vi "Przetwarzanie_szybkie_test.vi"() -> ()   [LabVIEW 2013]
uses:
  Kontrolki/Przetwarzanie/Kanaly.ctl
  Kontrolki/FVGs/FVG akwizycje akcje.ctl
  Kontrolki/FVGs/FVG akcje podstawowa.ctl
  <vilib>/measure/NI_MABase.lvlib
panel:
  in  "#cores (1)":i32=1
  out "szybka czasy":u32[](array[numeric])
  out "œrednia (ms)":dbl
  in  "stop":bool
  in  "L kanalow":i32=4
  out "Szybka":waveform(dbl)[](graph)
  in  "Szybka ZAKONCZ":bool
  out "Slide":dbl(slide)
  in  "Probki do usr":i32
  in  "#Cores (1)":i32=1
  out "# elements in queue":i32
  out "szybka czas":u32
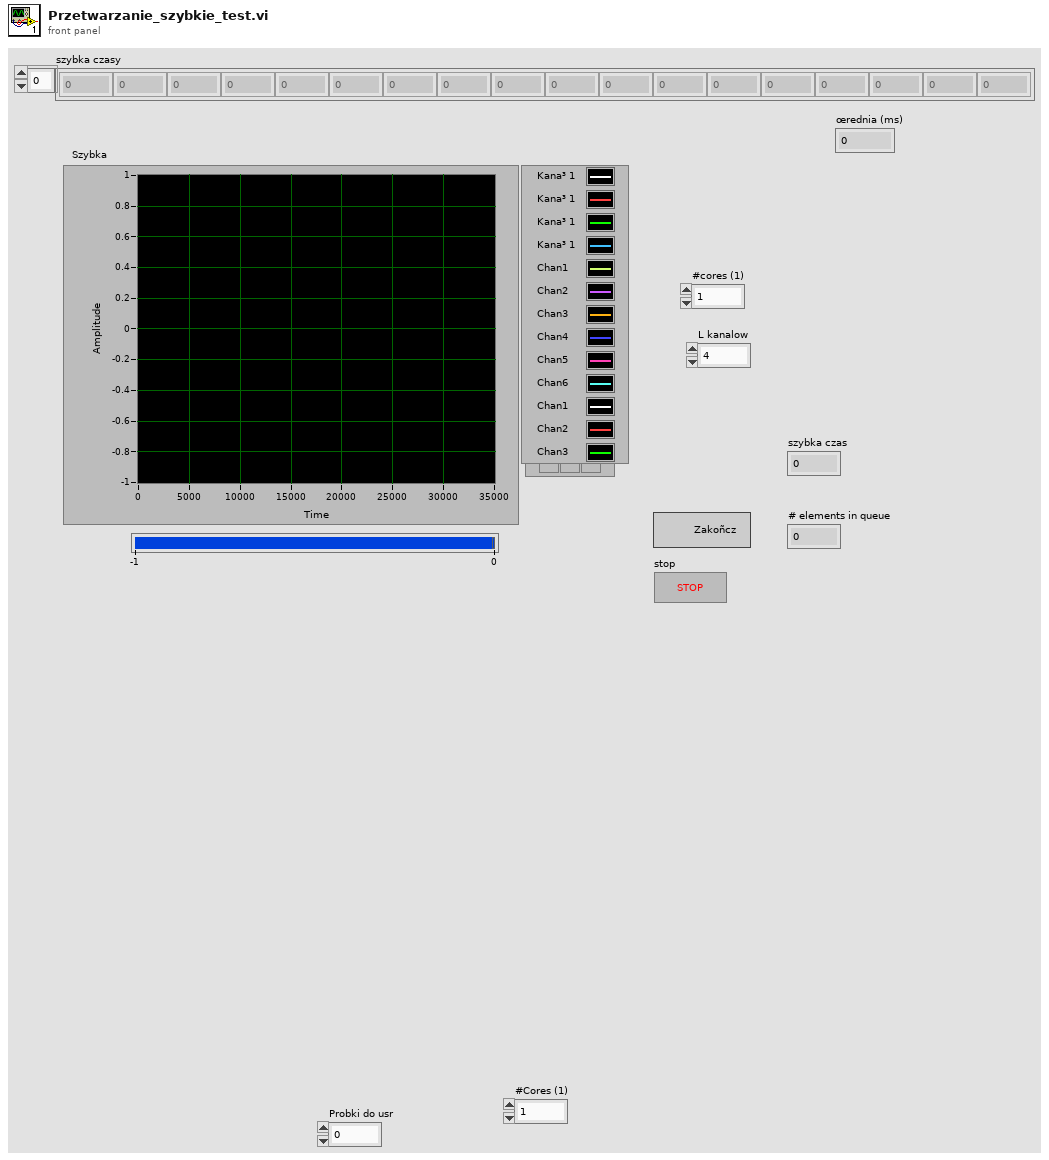
[diagram p1: front panel]
types:
  T1 = typedef "FVG akcje podstawowa.ctl" = enum16{"GET", "SET"}
  T2 = typedef "FVG akwizycje akcje.ctl" = enum16{"GET", "GETr", "SET"}
  T3 = typedef "Kanaly.ctl" = cluster{"Analogowe":waveform(dbl)[], "Cyfrowe":waveform(dbl)[], "Zwarcie":waveform(dbl)[], "Enkoder":waveform(dbl)[]}
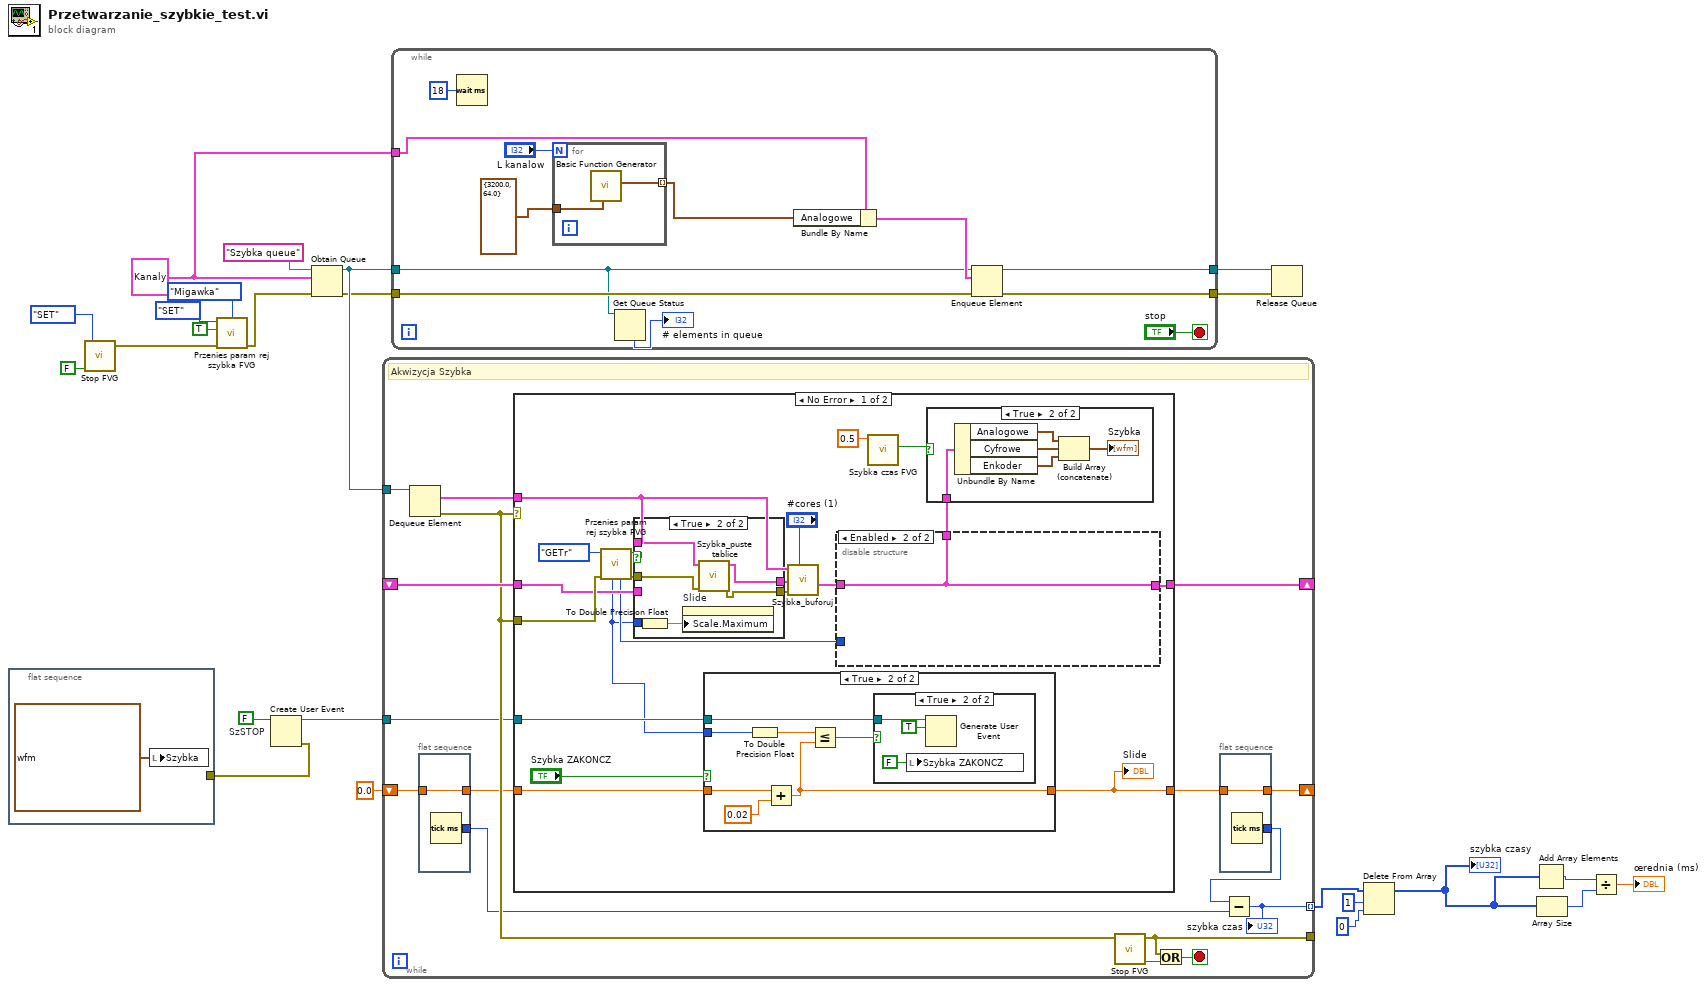
[diagram p0: block diagram]
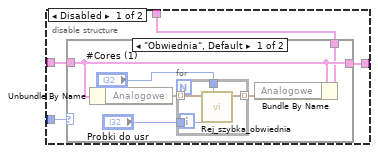
[diagram p3: hidden frame]
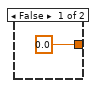
[diagram p6: hidden frame]
diagram:
  w21 = FALSE  # SzSTOP
  w22 = T3 data[32432B] ("Kanaly")
  n1 = flat-sequence {
    tunnel: w2 -> [_]
    frame #0 {
      n2 = local write "Szybka"(waveform(dbl)[] [{"t0"=timestamp(0 s since 1904-01-01), "dt"=1.0, "Y"=array[32000 elements]}, {"t0"=timestamp(0 s since 1904-01-01), "dt"=1.0, "Y"=array[32000 elements]}, {"t0"=timestamp(0 s since 1904-01-01), "dt"=1.0, "Y"=array[32000 elements]}, {"t0"=timestamp(0 s since 1904-01-01), "dt"=1.0, "Y"=array[32000 elements]}, {"t0"=timestamp(3504948842.5103908 s since 1904-01-01), "dt"=0.0003125, "Y"=array[8960 elements], "attributes"=variant("NI_ChannelName"=variant(string "Chan1"), "NI_UnitDescription"=variant(string "Volts"))}, {"t0"=timestamp(3504948842.5104046 s since 1904-01-01), "dt"=0.0003125, "Y"=array[8960 elements], "attributes"=variant("NI_ChannelName"=variant(string "Chan2"), "NI_UnitDescription"=variant(string "Volts"))}, {"t0"=timestamp(3504948842.510419 s since 1904-01-01), "dt"=0.0003125, "Y"=array[8960 elements], "attributes"=variant("NI_ChannelName"=variant(string "Chan3"), "NI_UnitDescription"=variant(string "Volts"))}, {"t0"=timestamp(3504948842.5104327 s since 1904-01-01), "dt"=0.0003125, "Y"=array[8960 elements], "attributes"=variant("NI_ChannelName"=variant(string "Chan4"), "NI_UnitDescription"=variant(string "Volts"))}, {"t0"=timestamp(3504948842.5104465 s since 1904-01-01), "dt"=0.0003125, "Y"=array[8960 elements], "attributes"=variant("NI_ChannelName"=variant(string "Chan5"), "NI_UnitDescription"=variant(string "Volts"))}, {"t0"=timestamp(3504948842.510461 s since 1904-01-01), "dt"=0.0003125, "Y"=array[8960 elements], "attributes"=variant("NI_ChannelName"=variant(string "Chan6"), "NI_UnitDescription"=variant(string "Volts"))}, {"t0"=timestamp(3504948842.5104747 s since 1904-01-01), "dt"=0.0003125, "Y"=array[8960 elements], "attributes"=variant("NI_ChannelName"=variant(string "Chan7"), "NI_UnitDescription"=variant(string "Volts"))}, {"t0"=timestamp(3504948842.5104885 s since 1904-01-01), "dt"=0.0003125, "Y"=array[8960 elements], "attributes"=variant("NI_ChannelName"=variant(string "Chan8"), "NI_UnitDescription"=variant(string "Volts"))}, {"t0"=timestamp(3504948842.510503 s since 1904-01-01), "dt"=0.0003125, "Y"=array[8960 elements], "attributes"=variant("NI_ChannelName"=variant(string "Digit1"), "NI_UnitDescription"=variant(string "Volts"))}, {"t0"=timestamp(3504948842.5105166 s since 1904-01-01), "dt"=0.0003125, "Y"=array[8960 elements], "attributes"=variant("NI_ChannelName"=variant(string "Digit2"), "NI_UnitDescription"=variant(string "Volts"))}, {"t0"=timestamp(3504948842.510531 s since 1904-01-01), "dt"=0.0003125, "Y"=array[8960 elements], "attributes"=variant("NI_ChannelName"=variant(string "Digit3"), "NI_UnitDescription"=variant(string "Volts"))}, {"t0"=timestamp(3504948842.510545 s since 1904-01-01), "dt"=0.0003125, "Y"=array[8960 elements], "attributes"=variant("NI_ChannelName"=variant(string "Digit4"), "NI_UnitDescription"=variant(string "Volts"))}, {"t0"=timestamp(3504948842.5103908 s since 1904-01-01), "dt"=0.0003125, "Y"=array[500 elements], "attributes"=variant("NI_ChannelName"=variant(string "Chan1"), "NI_UnitDescription"=variant(string "Volts"))}, {"t0"=timestamp(3504948842.5104046 s since 1904-01-01), "dt"=0.0003125, "Y"=array[500 elements], "attributes"=variant("NI_ChannelName"=variant(string "Chan2"), "NI_UnitDescription"=variant(string "Volts"))}, {"t0"=timestamp(3504948842.510419 s since 1904-01-01), "dt"=0.0003125, "Y"=array[500 elements], "attributes"=variant("NI_ChannelName"=variant(string "Chan3"), "NI_UnitDescription"=variant(string "Volts"))}, {"t0"=timestamp(3504948842.5104327 s since 1904-01-01), "dt"=0.0003125, "Y"=array[500 elements], "attributes"=variant("NI_ChannelName"=variant(string "Chan4"), "NI_UnitDescription"=variant(string "Volts"))}, {"t0"=timestamp(3504948842.5104465 s since 1904-01-01), "dt"=0.0003125, "Y"=array[500 elements], "attributes"=variant("NI_ChannelName"=variant(string "Chan5"), "NI_UnitDescription"=variant(string "Volts"))}, {"t0"=timestamp(3504948842.510461 s since 1904-01-01), "dt"=0.0003125, "Y"=array[500 elements], "attributes"=variant("NI_ChannelName"=variant(string "Chan6"), "NI_UnitDescription"=variant(string "Volts"))}, {"t0"=timestamp(3504948842.5104747 s since 1904-01-01), "dt"=0.0003125, "Y"=array[500 elements], "attributes"=variant("NI_ChannelName"=variant(string "Chan7"), "NI_UnitDescription"=variant(string "Volts"))}, {"t0"=timestamp(3504948842.5104885 s since 1904-01-01), "dt"=0.0003125, "Y"=array[500 elements], "attributes"=variant("NI_ChannelName"=variant(string "Chan8"), "NI_UnitDescription"=variant(string "Volts"))}, {"t0"=timestamp(3504948842.510503 s since 1904-01-01), "dt"=0.0003125, "Y"=array[500 elements], "attributes"=variant("NI_ChannelName"=variant(string "Digit1"), "NI_UnitDescription"=variant(string "Volts"))}, {"t0"=timestamp(3504948842.5105166 s since 1904-01-01), "dt"=0.0003125, "Y"=array[500 elements], "attributes"=variant("NI_ChannelName"=variant(string "Digit2"), "NI_UnitDescription"=variant(string "Volts"))}, {"t0"=timestamp(3504948842.510531 s since 1904-01-01), "dt"=0.0003125, "Y"=array[500 elements], "attributes"=variant("NI_ChannelName"=variant(string "Digit3"), "NI_UnitDescription"=variant(string "Volts"))}, {"t0"=timestamp(3504948842.510545 s since 1904-01-01), "dt"=0.0003125, "Y"=array[500 elements], "attributes"=variant("NI_ChannelName"=variant(string "Digit4"), "NI_UnitDescription"=variant(string "Volts"))}] ("Szybka")) -> ()
    }
  }
  n3 = call "Stop FVG.vi"("Akcja (GET)"=FVG_akcje_podstawowa."SET", "Stop in (F)"=FALSE) -> ("error out"=w6:errorcluster)  [unwired: 8 in, 1 out]
  n4 = call "Przenies param rej szybka FVG.vi"("Œledzenie In"=enum16{"Obwiednia", "Migawka"}."Migawka", "error in (no error)"=w6, "Start In"=TRUE, "Akcja"=FVG_akwizycje_akcje."SET") -> ("error out"=w9:errorcluster)  [unwired: 3 in, 4 out]
  n5 = Create User Event(user event datatype=w21) -> (user event=w20:refnum<user-event>, error out=w2:errorcluster)  [unwired: 1 in]
  n6 = Obtain Queue(name (unnamed)="Szybka queue", element data type=w22, error in (no error)=w9) -> (queue out=w23:refnum<queue>, error out=w19:errorcluster)  [unwired: 2 in, 1 out]
  n7 = while {
    tunnel: w23 -> [w41]
    tunnel: [w26] -> _
    shift-right: [w37] -> _
    shift-left: _ -> [w36]
    shift-right: [w32] -> _
    shift-left: 0.0 -> [w31]
    tunnel: w20 -> [w34]
    tunnel: [w27] -> w10 mode=indexing
    stop <- w39 stop-if-true
    # "Akwizycja Szybka"
    n8 = Dequeue Element(queue=w41) -> (element=w38:T3, error out=w35:errorcluster)  [unwired: 2 in, 2 out]
    n9 = flat-sequence {
      tunnel: w31 -> [w43]
      tunnel: [w43] -> w30
      tunnel: [w42] -> w29
      frame #0 {
        n10 = Tick Count (ms)() -> (millisecond timer value=w42:u32)
      }
    }
    n11 = case shown="No Error" w35 {
      tunnel: w38 -> [w56 _]
      tunnel: [w52 w107] -> w37
      tunnel: w36 -> [w58 w107]
      tunnel: w35 -> [w64 _]
      tunnel: w30 -> [w62 w106]
      tunnel: [w61 w106] -> w33
      tunnel: w34 -> [w60 _]
      frame No Error {
        n12 = call "Przenies param rej szybka FVG.vi"("error in (no error)"=w64, "Akcja"=FVG_akwizycje_akcje."GETr") -> ("error out"=w55:errorcluster, "Restart Out"=w59:bool, "Œledzenie Out"=w51:enum16{"Obwiednia", "Migawka"}, "Czas Out"=w46:i32)  [unwired: 5 in, 1 out]
        n13 = case shown="True" w59 {
          tunnel: w58 -> [w88 _]
          tunnel: [w88 w93] -> w57
          tunnel: w56 -> [_ w94]
          tunnel: w55 -> [w87 w92]
          tunnel: [w87 w91] -> w54
          tunnel: w46 -> [_ w89]
          frame False {
          }
          frame True {
            n14 = To Double Precision Float(number=w89) -> (double precision float=w90:dbl)
            n15 = property on="Slide" class="Slide (strict)"("Scale.Maximum"=w90) -> ()  [unwired: 2 in, 2 out]
            n16 = call "Szybka_puste tablice.vi"("error in (no error)"=w92, "Kanaly in"=w94) -> ("error out"=w91:errorcluster, "Kanaly out"=w93:T3)  [unwired: 8 in]
          }
        }
        n17 = case shown="True" "Szybka ZAKONCZ" {
          tunnel: w62 -> [_ w101]
          tunnel: [0.0 w98] -> w61
          tunnel: w46 -> [_ w100]
          tunnel: w60 -> [_ w96]
          frame False {
          }
          frame True {
            n18 = To Double Precision Float(number=w100) -> (double precision float=w99:dbl)
            n19 = Add(x=w101, y=0.02) -> (x+y=w98:dbl)
            n20 = Less Or Equal?(x=w99, y=w98) -> (x <= y?=w97:bool)
            n21 = case shown="True" w97 {
              tunnel: w96 -> [_ w104]
              frame False {
              }
              frame True {
                n22 = local write "Szybka ZAKONCZ"(FALSE ("Szybka ZAKONCZ")) -> ()
                n23 = Generate User Event(user event=w104, event data cluster=TRUE ("event data")) -> ()  [unwired: 2 in, 2 out]
              }
            }
          }
        }
        "Slide" <- w61
        n24 = call "Szybka_buforuj.vi"("#cores (1)"="#cores (1)", "error in (no error)"=w54, "Bufor in"=w57, "Kanaly in"=w56) -> ("Bufor out"=w53:T3)  [unwired: 6 in, 1 out]
        n25 = disable-structure shown="Enabled" {
          disable-tunnel: w53 -> [w74 w86]
          disable-tunnel: [w73 w86] -> w52
          disable-tunnel: w51 -> [w72 _]
          disable-tunnel: [w71 w86] -> w50
          frame Disabled {
            n26 = case shown="\"Obwiednia\", Default" w72 {
              tunnel: w74 -> [w76 w85]
              tunnel: [w76 w85] -> w73
              tunnel: [w75 w85] -> w71
              frame "Obwiednia", Default {
                n27 = Unbundle By Name(w76) -> ("Analogowe"=w80:waveform(dbl)[])
                n28 = for {
                  tunnel: w80 -> [w84] mode=indexing
                  tunnel: [w83] -> w79 mode=indexing
                  tunnel: "Probki do usr" -> [w82]
                  tunnel: "#Cores (1)" -> [w81]
                  n29 = call "Rej_szybka_obwiednia.vi"("Liczba probek (200)"=w82, "#Cores (1)"=w81, "Wfm in"=w84) -> ("Wfm max out"=w83:waveform(dbl))  [unwired: 6 in, 2 out]
                }
                n30 = Bundle By Name(cluster=w76, "Analogowe"=w79) -> (w75:T3)
              }
              frame "Migawka" {
              }
            }
          }
          frame Enabled {
          }
        }
        n31 = call "Szybka czas FVG.vi"("Zadany"=0.5) -> ("Elapsed?"=w47:bool)  [unwired: 9 in, 1 out]
        n32 = case shown="True" w47 {
          tunnel: w50 -> [_ w66]
          frame False {
          }
          frame True {
            n33 = Unbundle By Name(w66) -> ("Analogowe"=w70:waveform(dbl)[], "Cyfrowe"=w69:waveform(dbl)[], "Enkoder"=w68:waveform(dbl)[])
            n34 = Build Array (concatenate)(w70, w69, w68) -> (→"Szybka":waveform(dbl)[])
          }
        }
      }
      frame Error {
      }
    }
    n35 = call "Stop FVG.vi"("error in (no error)"=w35) -> ("Stop out"=w40:bool, "error out"=w26:errorcluster)  [unwired: 9 in]
    n36 = Or(x=w26, y=w40) -> (x .or. y?=w39:bool)
    n37 = flat-sequence {
      tunnel: w33 -> [w45]
      tunnel: [w45] -> w32
      tunnel: [w44] -> w28
      frame #0 {
        n38 = Tick Count (ms)() -> (millisecond timer value=w44:u32)
      }
    }
    n39 = Subtract(x=w28, y=w29) -> (x-y=w27:u32)
    "szybka czas" <- w27
  }
  n40 = while {
    tunnel: w23 -> [w109]
    tunnel: w22 -> [w117]
    tunnel: w19 -> [w114]
    tunnel: [w113] -> w18
    tunnel: [w112] -> w17
    stop <- "stop" stop-if-true
    n41 = Wait (ms)(milliseconds to wait=u32 18) -> ()  [unwired: 1 out]
    n42 = for {
      N: "L kanalow" -> [_]
      tunnel: [w121] -> w116 mode=indexing
      tunnel: cluster{"Fs":dbl, "#s":dbl} {"Fs"=3200.0, "#s"=64.0} ("sampling info") -> [w120]
      n43 = call <vilib>:"Basic Function Generator.vi"("sampling info"=w120) -> ("signal out"=w121:waveform(dbl))  [unwired: 8 in, 2 out]
    }
    n44 = Get Queue Status(queue=w109) -> (# elements in queue=→"# elements in queue":i32)  [unwired: 2 in, 7 out]
    n45 = Bundle By Name(cluster=w117, "Analogowe"=w116) -> (w115:T3)
    n46 = Enqueue Element(queue=w109, element=w115, error in (no error)=w114) -> (queue out=w113:refnum<queue>, error out=w112:errorcluster)  [unwired: 1 in, 1 out]
  }
  n47 = Release Queue(queue=w18, error in (no error)=w17) -> ()  [unwired: 1 in, 3 out]
  n48 = Delete From Array(array=w10, length=1, index=0) -> (array with subset deleted=w14:u32[])  [unwired: 1 out]
  "szybka czasy" <- w14
  n49 = Add Array Elements(numeric array=w14) -> (sum=w12:u32)
  n50 = Array Size(array=w14) -> (size(s)=w11:i32)
  n51 = Divide(x=w12, y=w11) -> (x/y=→"œrednia (ms)":dbl)
